vi "Window Position Set.vi"(4 "window refnum":T1, 5 "error in (no error)":errorcluster, 6 "activate error message? (T)":bool=TRUE, 7 "activate window? (T)":bool=TRUE, 8 "window position":i16(ring) items=["Not Topmost", "Topmost", "Top", "Bottom"]) -> (0 "error out":errorcluster)   [LabVIEW 2017]
doc: "This VI will set the position of a window identified by the 'window refnum'."
uses:
  <vilib>/ExportToExcel/Window Refnum.ctl
  user32.dll
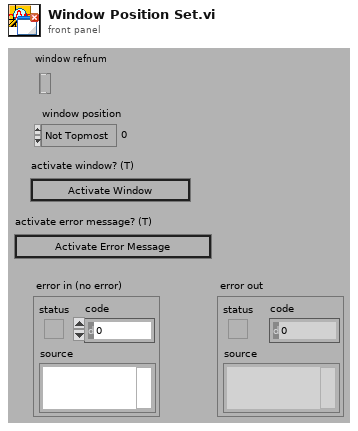
[diagram p1: front panel]
types:
  T1 = typedef "Window Refnum.ctl" = refnum<k1>
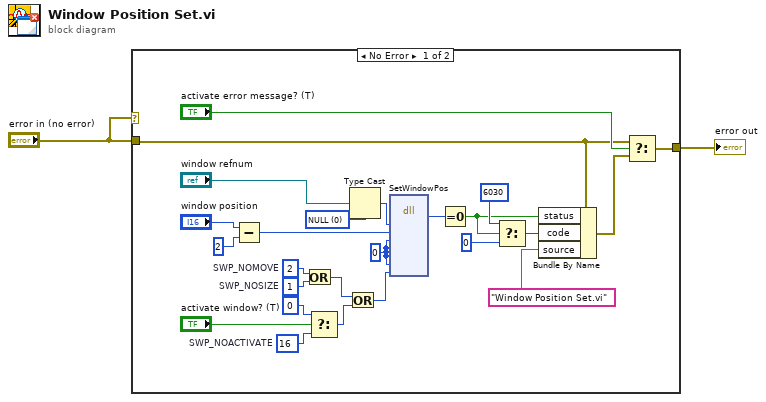
[diagram p0: block diagram]
diagram:
  n1 = case shown="No Error" "error in (no error)" {
    tunnel: "error in (no error)" -> [w4 w28]
    tunnel: [w6 w28] -> w1
    frame No Error {
      w19 = u32 2  # SWP_NOMOVE
      w20 = u32 1  # SWP_NOSIZE
      w22 = u32 16  # SWP_NOACTIVATE
      w15 = u32 0 items=["NULL"]
      w27 = 0
      n2 = Subtract(x="window position", y=i16 2) -> (x-y=w18:i16)
      n3 = Or(x=w19, y=w20) -> (x .or. y?=w25:u32)
      n4 = Select(t=u32 0, s="activate window? (T)", f=w22) -> (s? t:f=w24:u32)
      n5 = Or(x=w25, y=w24) -> (x .or. y?=w26:u32)
      n6 = Type Cast(type=w15, x="window refnum") -> (*(type *) &x=w16:u32)
      n7 = dll-call lib="user32.dll" fn="SetWindowPos"("hWnd"=w16, "hWndInsertAfter"=w18, "left"=w27, "top"=w27, "width"=w27, "height"=w27, "fuFlags"=w26) -> ("error"=w13:i32)  [unwired: 10 in, 2 out]
      n8 = Equal To 0?(x=w13) -> (x = 0?=w8:bool)
      n9 = Select(t=6030, s=w8, f=0) -> (s? t:f=w9:i32)
      n10 = Bundle By Name(cluster=w4, "status"=w8, "code"=w9, "source"="Window Position Set.vi") -> (w3:errorcluster)
      n11 = Select(t=w4, s="activate error message? (T)", f=w3) -> (s? t:f=w6:errorcluster)
    }
    frame Error {
    }
  }
  "error out" <- w1
